vi "StopMeasurement.vi"(8 "error in (no error)":errorcluster, 11 "Multiharp in":refnum<class "Multiharp.lvclass">) -> (0 "error out":errorcluster, 3 "Multiharp out":refnum<class "Multiharp.lvclass">)   [LabVIEW 2023, in "SinglePhoton Library.lvlib" / "Multiharp.lvlib" / "Multiharp.lvclass"]
uses:
  Multiharp.lvclass
  Multiharp.lvclass/Multiharp.ctl
panel:
  in  "event data":T1
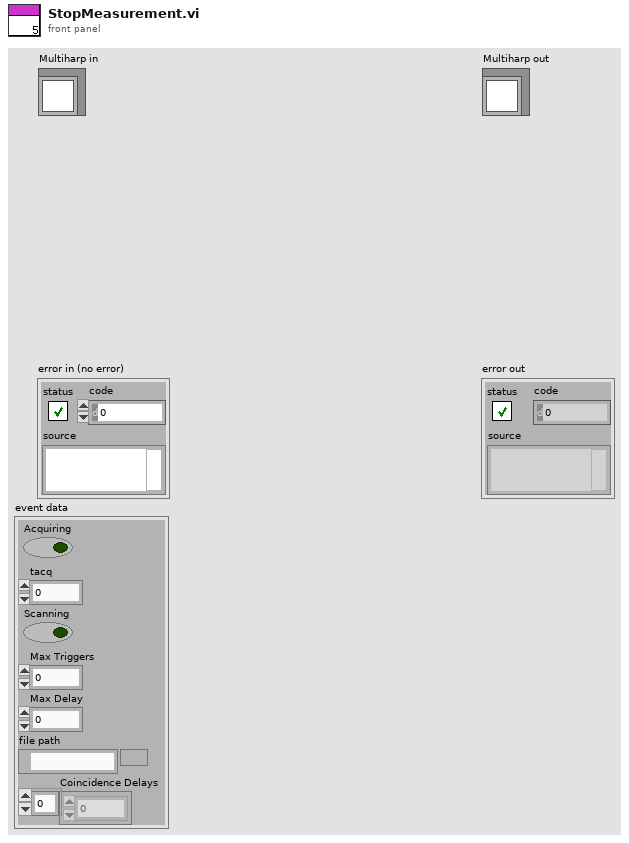
[diagram p1: front panel]
types:
  T1 = cluster{"Acquiring":bool, "tacq":i32, "Scanning":bool, "Max Triggers":i32, "Max Delay":dbl, "file path":path, "Coincidence Delays":dbl[]}
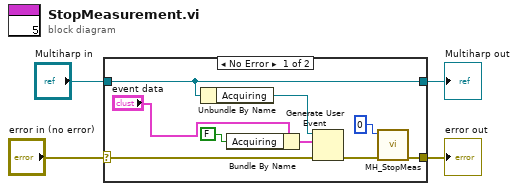
[diagram p0: block diagram]
diagram:
  n1 = case shown="No Error" "error in (no error)" {
    selector: "error in (no error)" -> [w9 w15]
    tunnel: [w10 w15] -> w3
    tunnel: [w12 w14] -> w1
    tunnel: "Multiharp in" -> [w12 w14]
    frame No Error {
      n2 = Unbundle By Name(w12) -> ("Acquiring"=w13:refnum<user-event>)
      n3 = Bundle By Name(cluster="event data", "Acquiring"=FALSE) -> (w6:T1)
      n4 = Generate User Event(user event=w13, event data cluster=w6, error in=w9) -> (error out=w11:errorcluster)  [unwired: 1 in, 1 out]
      n5 = call "MH_StopMeas.vi"("error in (no error)"=w11, "devidx"=0) -> ("error out"=w10:errorcluster)  [unwired: 8 in, 1 out]
    }
    frame Error {
    }
  }
  "error out" <- w3
  "Multiharp out" <- w1
